vi "create_new_lifo_svi.vi"(8 "error in (no error)":errorcluster, 10 "Name in":string) -> (0 "error out":errorcluster, 1 "Key Index":i32, 2 "Name Out":string)   [LabVIEW 2015]
uses:
  index_cluster.ctl
  C:/Users/Giuseppe/Downloads/LabLinda_ pakage/index_datatype.ctl
  C:/Users/Giuseppe/Downloads/LabLinda_ pakage/index_cluster.ctl
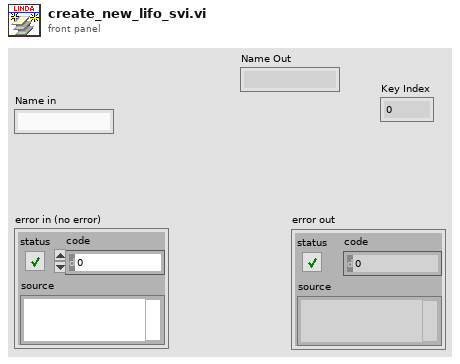
[diagram p1: front panel]
types:
  T1 = typedef "index_cluster.ctl" = cluster{"Addr":i32[], "out react vi reference":refnum<vi>, "in react vi reference":refnum<vi>, "rd react vi reference":refnum<vi>, "Read_write_var":refnum<vi>}
  T2 = typedef "index_datatype.ctl" = T1[]
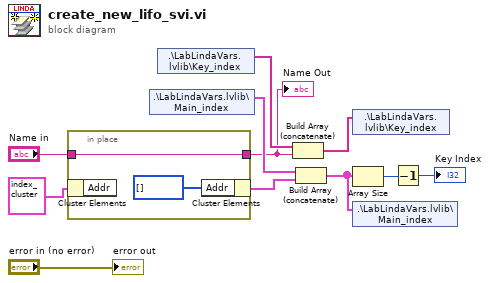
[diagram p0: block diagram]
diagram:
  n1 = in-place {
    in-place-border: "Name in" -> [w13]
    in-place-border: [w13] -> w1
    n2 = in-place-cluster #1(T1 {"Addr"=[], "out react vi reference"=refnum, "in react vi reference"=refnum, "rd react vi reference"=refnum, "Read_write_var"=refnum} ("index_cluster")) -> ()  [unwired: 1 out]
    n3 = in-place-cluster #1("Addr"=i32[] []) -> (w10:T1)
  }
  "Name Out" <- w1
  n4 = shared-variable ".\\LabLindaVars.lvlib\\Main_index"() -> (w11:T2)  [unwired: 1 in, 1 out]
  n5 = shared-variable ".\\LabLindaVars.lvlib\\Key_index"() -> (w9:string[])  [unwired: 1 in, 1 out]
  n6 = Build Array (concatenate)(w9, w1) -> (w6:string[])
  n7 = Build Array (concatenate)(w11, w10) -> (w5:T2)
  n8 = shared-variable ".\\LabLindaVars.lvlib\\Key_index"(w6) -> ()  [unwired: 1 in, 1 out]
  n9 = Array Size(array=w5) -> (size(s)=w4:i32)
  n10 = shared-variable ".\\LabLindaVars.lvlib\\Main_index"(w5) -> ()  [unwired: 1 in, 1 out]
  n11 = Decrement(x=w4) -> (x-1=→"Key Index":i32)
  "error out" <- "error in (no error)"
